vi "Disarm.vi"(8 "error in (no error)":errorcluster, 9 "Request type":T1, 10 "Requester":string, 11 "Lockin Digitizer in":refnum<class "Lockin Digitizer.lvclass">) -> (0 "error out":errorcluster, 3 "Lockin Digitizer out":refnum<class "Lockin Digitizer.lvclass">)   [LabVIEW 2021, in "Lockin Digitizer.lvclass"]
uses:
  Lockin Digitizer.lvclass
  C:/Program Files/National Instruments/LabVIEW 2021/vi.lib/ActorFramework/Actor/Actor.lvclass
  Controllers/Process Controller/Request type.ctl
  Lockin Digitizer Messages/Lock-in Command Msg/Lock-in Command Msg.lvclass
  C:/Program Files/National Instruments/LabVIEW 2021/vi.lib/ActorFramework/Message/Message.lvclass
  <vilib>/ActorFramework/Actor/Actor.lvclass/Actor.ctl
  <vilib>/ActorFramework/Message Enqueuer/Message Enqueuer.lvclass/Message Enqueuer.ctl
  <vilib>/ActorFramework/Message Enqueuer/Init from Existing Queue.vi
  NHMFL_Core/Libraries/Instruments/Pulse Driver/Lockin Digitizer Driver/Lockin Digitizer Driver.lvclass
  <vilib>/ActorFramework/Message Enqueuer/Message Enqueuer.lvclass
  Pulse Recorder Actor/Pulse Recorder Actor.lvclass
  Lockin Digitizer.lvclass/Lockin Digitizer.ctl
  <vilib>/ActorFramework/Actor/Actor.lvclass
  L-D Command Context.ctl
panel:
  out "Lockin active":bool
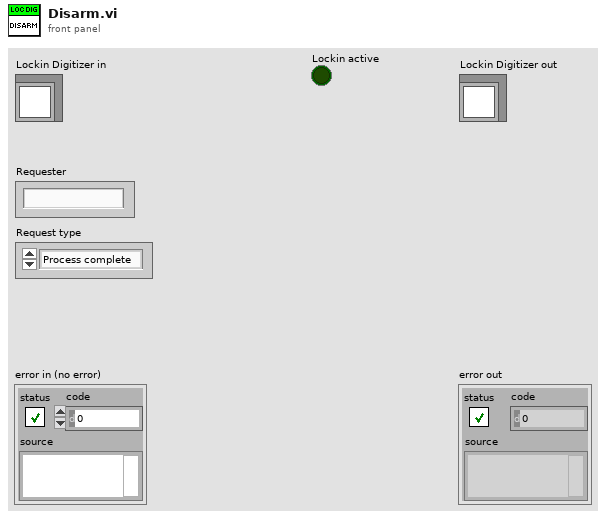
[diagram p1: front panel]
types:
  T1 = typedef "Request type.ctl" = enum16{"Process complete", "User command", "Auto-restart", "Error"}
  T2 = typedef "L-D Command Context.ctl" = enum16{"Re", "Switch", "Measure", "Arm"}
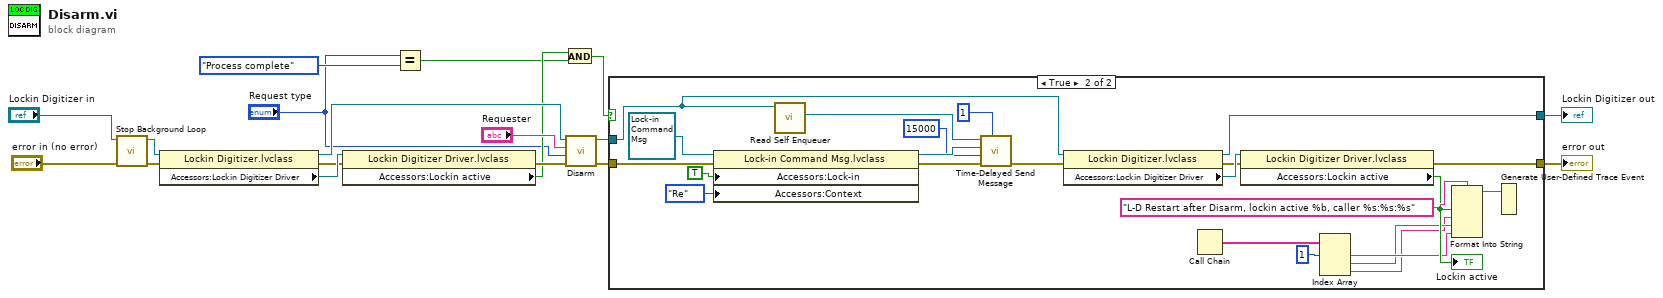
[diagram p0: block diagram]
diagram:
  n1 = call-dynamic "Stop Background Loop.vi"("error in (no error)"="error in (no error)", "Worker Actor in"="Lockin Digitizer in") -> ("error out"=w6:errorcluster, "Worker Actor out"=w4:refnum<class "Lockin Digitizer.lvclass">)  [unwired: 8 in]
  n2 = property class="Lockin Digitizer.lvclass"(reference=w4, error in=w6) -> (reference out=w17:refnum<class "Lockin Digitizer.lvclass">, error out=w15:errorcluster, "Accessors:Lockin Digitizer Driver"=w16:refnum<class "Lockin Digitizer Driver.lvclass">)
  n3 = property class="Lockin Digitizer Driver.lvclass"(reference=w16, error in=w15) -> (error out=w14:errorcluster, "Accessors:Lockin active"=w10:bool)  [unwired: 1 out]
  n4 = Equal?(x="Request type", y=Request_type."Process complete") -> (x = y?=w8:bool)
  n5 = And(x=w10, y=w8) -> (x .and. y?=w11:bool)
  n6 = call-parent "Disarm.vi"("error in (no error)"=w14, "Request type"="Request type", "Requester"="Requester", "Pulse Recorder Actor in"=w17) -> ("error out"=w3:errorcluster, "Pulse Recorder Actor out"=w2:refnum<class "Lockin Digitizer.lvclass">)  [unwired: 6 in]
  n7 = case shown="True" w11 {
    tunnel: w3 -> [w19 w27]
    tunnel: w2 -> [w20 w35]
    tunnel: [w20 w36] -> w13
    tunnel: [w19 w29] -> w12
    frame False {
    }
    frame True {
      n8 = property class="Lock-in Command Msg.lvclass"(reference=refnum<class "Lock-in Command Msg.lvclass"> refnum ("Lock-in Command Msg.lvclass"), error in=w27, "Accessors:Lock-in"=TRUE ("Lock-in"), "Accessors:Context"=L-D_Command_Context."Re" ("Context")) -> (reference out=w42:refnum<class "Lock-in Command Msg.lvclass">, error out=w28:errorcluster)
      n9 = call <vilib>:"Read Self Enqueuer.vi"("Actor"=w35) -> ("Self Enqueuer"=w40:refnum<class "Message Enqueuer.lvclass">)  [unwired: 10 in]
      n10 = call <vilib>:"Time-Delayed Send Message.vi"("# Copies (0 = infinite repeat)"=u32 1, "error in (no error)"=w28, "Milliseconds To Wait"=15000, "Message"=w42, "Message Enqueuer"=w40) -> ("error out"=w34:errorcluster)  [unwired: 5 in, 1 out]
      n11 = property class="Lockin Digitizer.lvclass"(reference=w35, error in=w34) -> (reference out=w36:refnum<class "Lockin Digitizer.lvclass">, error out=w30:errorcluster, "Accessors:Lockin Digitizer Driver"=w37:refnum<class "Lockin Digitizer Driver.lvclass">)
      n12 = Call Chain() -> (call chain=w26:string[])
      n13 = property class="Lockin Digitizer Driver.lvclass"(reference=w37, error in=w30) -> (error out=w29:errorcluster, "Accessors:Lockin active"=w31:bool)  [unwired: 1 out]
      "Lockin active" <- w31
      n14 = Index Array(array=w26, index #1=1 ("index")) -> (element #1=w24:string, element #2=w23:string, element #3=w22:string)  [unwired: 2 in]
      n15 = Format Into String(format string="L-D Restart after Disarm, lockin active %b, caller %s:%s:%s" ("string"), w31, w22, w23, w24) -> (resulting string=w32:string)  [unwired: 2 in, 1 out]
      n16 = Generate User-Defined Trace Event(2:w32) -> ()  [unwired: 1 in]
    }
  }
  "error out" <- w12
  "Lockin Digitizer out" <- w13
